vi "Encode Key.vi"(9 "Pretty Indent (-1=None)":i32=-1, 10 "JSON Value":string, 11 "Key (\"\"=Value only)":string) -> (3 "JSON out":string)   [LabVIEW 2019, in "JSON.lvlib"]
uses:
  JSON.lvlib
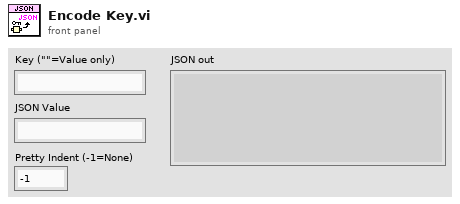
[diagram p1: front panel]
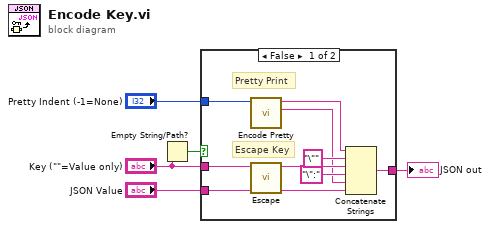
[diagram p0: block diagram]
diagram:
  n1 = Empty String/Path?(string/path="Key (\"\"=Value only)") -> (empty?=w5:bool)
  n2 = case shown="False" w5 {
    tunnel: "JSON Value" -> [w9 w15]
    tunnel: [w12 w15] -> w1
    tunnel: "Key (\"\"=Value only)" -> [w10 _]
    tunnel: "Pretty Indent (-1=None)" -> [w8 _]
    frame False {
      # "Pretty Print"
      # "Escape Key"
      n3 = call "Encode Pretty.vi"("Pretty Indent (-1=None)"=w8) -> ("key-value gap"=w6:string, "prefix"=w7:string)  [unwired: 8 in, 1 out]
      n4 = call "Escape.vi"("string"=w10) -> ("escaped string"=w11:string)  [unwired: 10 in]
      n5 = Concatenate Strings(w7, "\"" ("string"), w11, "\":" ("string"), w6, w9) -> (w12:string)
    }
    frame True {
      # "Empty Key \n== Return Value only"
    }
  }
  "JSON out" <- w1
